vi "mcc_usb202_read.vi"(6 "error in":errorcluster, 11 "task in":refnum<k24>) -> (0 "status":bool=TRUE, 1 "V1":dbl, 2 "V0":dbl, 3 "task out":refnum<k24>, 4 "error out":errorcluster={"status"=TRUE, "code"=10023, "source"="ULx Create Channel (AI-Voltage-Basic).vi:5780001<ERR>\nMeasurements: Channel not specified."})   [LabVIEW 2019]
uses:
  C:/Program Files/National Instruments/LabVIEW 2019/vi.lib/ULx/ULx_LV.dll
  Program Files/National Instruments/LabVIEW 2019/vi.lib/ULx/ULx_LV.dll
  <vilib>/Analysis/baseanly.llb/Mean (DBL).vi
  <vilib>/ULx/Read.llb/ULx Read (Analog 2D DBL NChan NSamp).vi
  <vilib>/Analysis/NI_AALBase.lvlib
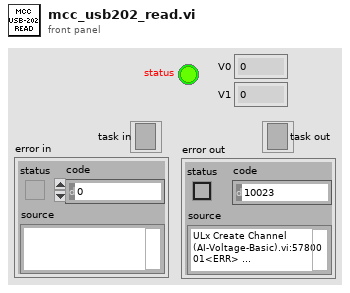
[diagram p1: front panel]
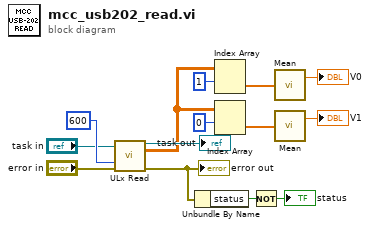
[diagram p0: block diagram]
diagram:
  n1 = call-poly <vilib>:"ULx Read.vi"("task in"="task in", "timeout"=600, "error in"="error in") -> ("task out"=→"task out":refnum<k24>, "data"=w5:dbl[][], "error out"=w10:errorcluster)  [unwired: 10 in]
  "error out" <- w10
  n2 = Unbundle By Name(w10) -> ("status"=w9:bool)
  n3 = Index Array(array=w5, index (row)=1 ("index")) -> (element=w4:dbl[])  [unwired: 1 in]
  n4 = Index Array(array=w5, index (row)=0 ("index")) -> (element=w2:dbl[])  [unwired: 1 in]
  n5 = Not(x=w9) -> (.not. x?=→"status":bool)
  n6 = call-poly <vilib>:"Mean.vi"("X"=w4) -> ("mean"=→"V0":dbl)  [unwired: 1 out]
  n7 = call-poly <vilib>:"Mean.vi"("X"=w2) -> ("mean"=→"V1":dbl)  [unwired: 1 out]
